vi "Load App.vi"(8 "error in (no error)":errorcluster, 11 "Status Notifier":refnum<notifier>) -> (0 "error out":errorcluster)   [LabVIEW 2018, in "Air Cooler Application.lvlib" / "Air Cooler Application.lvclass"]
doc: "Perform any work needed when loading the application. The input notifier is used to send text to the splash screen that will be displayed to the user. The text specifies what stage the load process is in."
uses:
  Air Cooler Application.lvclass
  C:/Program Files (x86)/National Instruments/LabVIEW 2018/vi.lib/ActorFramework/Actor/Actor.lvclass
  <vilib>/ActorFramework/Actor/Actor.lvclass
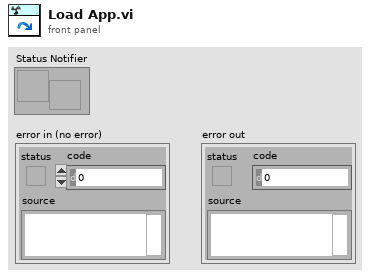
[diagram p1: front panel]
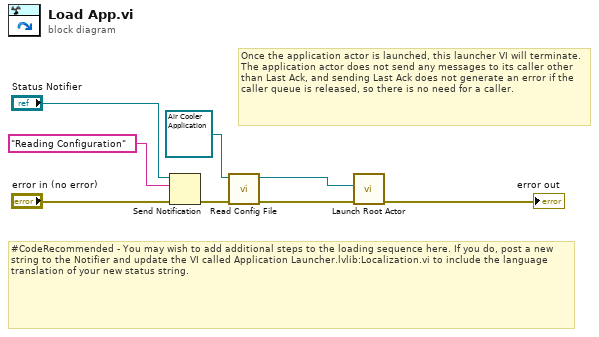
[diagram p0: block diagram]
diagram:
  # "Once the application actor is launched, this launcher VI will terminate. The application actor does not send any messages to its caller other than Last Ack, and sending Last Ack does not generate an error if the caller queue is released, so there is no need for a caller."
  # "#CodeRecommended - You may wish to add additional steps to the loading sequence here. If you do, post a new string to the Notifier and update the VI called Application Launcher.lvlib:Localization.vi to include the language translation of your new status string."
  n1 = Send Notification(notification="Reading Configuration", notifier="Status Notifier", error in (no error)="error in (no error)") -> (error out=w4:errorcluster)  [unwired: 1 out]
  n2 = call-dynamic "Read Config File.vi"("error in (no error)"=w4, "Air Cooler Application in"=refnum<class "Air Cooler Application.lvclass"> refnum ("My Application.lvclass")) -> ("error out"=w2:errorcluster, "Air Cooler Application out"=w1:refnum<class "Air Cooler Application.lvclass">)  [unwired: 8 in]
  n3 = call <vilib>:"Launch Root Actor.vi"("error in (no error)"=w2, "Actor"=w1) -> ("error out"=→"error out":errorcluster)  [unwired: 8 in, 1 out]
